vi "get_remaining_samples_to_read.vi"(8 "error in (no error)":errorcluster, 11 "GenericDAQ in":refnum<class "GenericDAQ.lvclass">) -> (0 "error out":errorcluster, 2 "remaining samples to read":i64, 3 "GenericDAQ out":refnum<class "GenericDAQ.lvclass">)   [LabVIEW 2010, in "GenericDAQ.lvclass"]
uses:
  GenericDAQ.lvclass
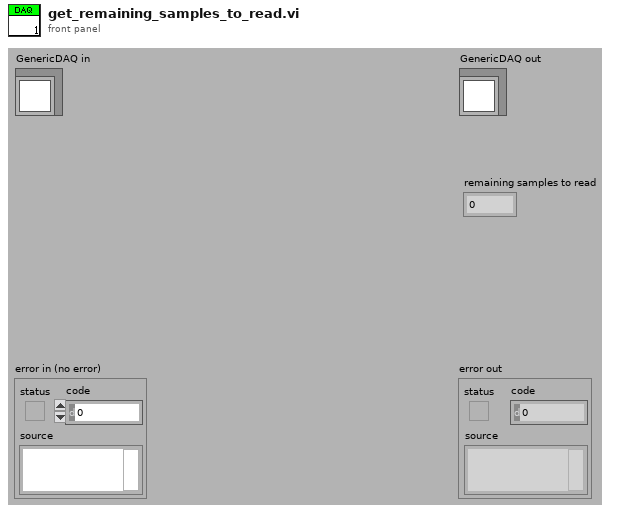
[diagram p1: front panel]
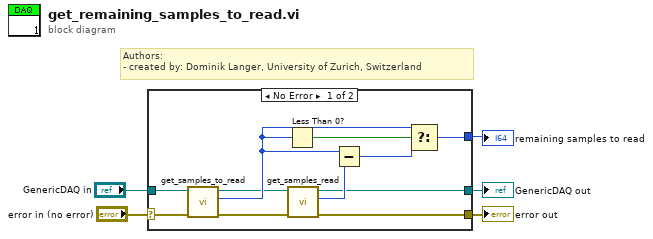
[diagram p0: block diagram]
diagram:
  # "Authors: \n- created by: Dominik Langer, University of Zurich, Switzerland"
  n1 = case shown="No Error" "error in (no error)" {
    selector: "error in (no error)" -> [w16 w18]
    tunnel: [w8 w18] -> w4
    tunnel: [w10 w17] -> w2
    tunnel: "GenericDAQ in" -> [w15 w17]
    tunnel: [w6 _] -> w1
    frame No Error {
      n2 = call-dynamic "get_samples_to_read.vi"("error in (no error)"=w16, "GenericDAQ.lvclass in"=w15) -> ("error out"=w9:errorcluster, "samples to read"=w12:i64, "GenericDAQ.lvclass out"=w11:refnum<class "GenericDAQ.lvclass">)  [unwired: 7 out]
      n3 = Less Than 0?(x=w12) -> (x < 0?=w14:bool)
      n4 = call-dynamic "get_samples_read.vi"("error in (no error)"=w9, "GenericDAQ.lvclass in"=w11) -> ("error out"=w8:errorcluster, "samples read"=w13:i64, "GenericDAQ.lvclass out"=w10:refnum<class "GenericDAQ.lvclass">)  [unwired: 7 out]
      n5 = Subtract(x=w12, y=w13) -> (x-y=w7:i64)
      n6 = Select(t=w12, s=w14, f=w7) -> (s? t:f=w6:i64)
    }
    frame Error {
    }
  }
  "error out" <- w4
  "GenericDAQ out" <- w2
  "remaining samples to read" <- w1
